vi "Attempt Repair.vi"(8 "error in":errorcluster, 11 "NISE_CEF_serializable node in":refnum<class "NISE_CEF_serializable node.lvclass">) -> (0 "error out":errorcluster, 2 "refresh tree?":bool, 3 "NISE_CEF_serializable node out":refnum<class "NISE_CEF_serializable node.lvclass">)   [LabVIEW 2013, in "NISE_CEF_serializable node.lvclass"]
uses:
  NISE_CEF_serializable node.lvclass
  serializable configuration/NISE_CEF_serializable configuration.lvclass
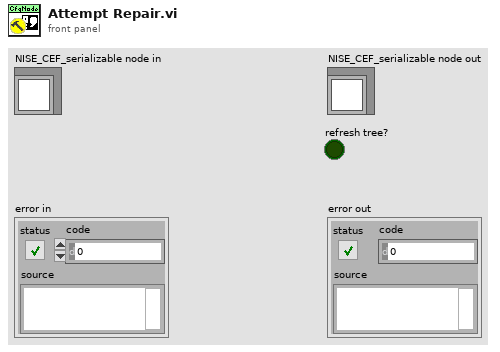
[diagram p1: front panel]
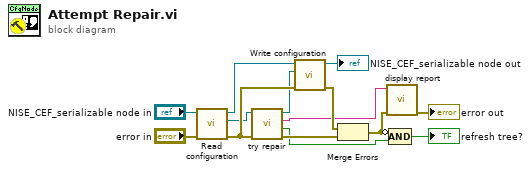
[diagram p0: block diagram]
diagram:
  n1 = call-dynamic "Read configuration.vi"("error in"="error in", "NISE_CEF_serializable node in"="NISE_CEF_serializable node in") -> ("error out"=w9:errorcluster, "configuration"=w8:refnum<class "NISE_CEF_serializable configuration.lvclass">, "NISE_CEF_serializable node out"=w6:refnum<class "NISE_CEF_serializable node.lvclass">)  [unwired: 7 in]
  n2 = call "try repair.vi"("error in"=w9, "configuration in"=w8) -> ("error out"=w10:errorcluster, "change occurred"=w5:bool, "repair report"=w1:string, "configuration out"=w7:refnum<class "NISE_CEF_serializable configuration.lvclass">)  [unwired: 6 in]
  n3 = call-dynamic "Write configuration.vi"("error in"=w9, "configuration"=w7, "NISE_CEF_serializable node in"=w6) -> ("error out"=w11:errorcluster, "NISE_CEF_serializable node out"=→"NISE_CEF_serializable node out":refnum<class "NISE_CEF_serializable node.lvclass">)  [unwired: 7 in]
  n4 = Merge Errors(w11, w10) -> (w2:errorcluster)
  n5 = call "display report.vi"("error in"=w2, "data to display"=w1) -> ("error out"=→"error out":errorcluster)  [unwired: 9 in]
  n6 = Compound Arithmetic op=AND(invert w2, w5) -> (→"refresh tree?":bool)
